vi "Parse RANGEFINDER.vi"(11 "Data":string) -> (2 "Voltage":sgl, 3 "Distance (m)":sgl)   [LabVIEW 2014]
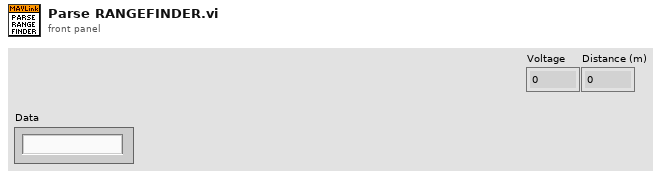
[diagram p1: front panel]
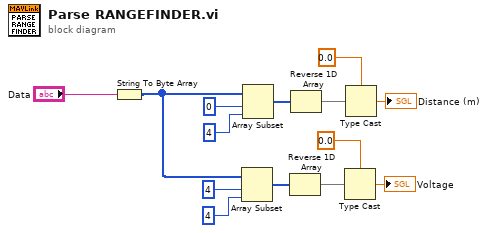
[diagram p0: block diagram]
diagram:
  n1 = String To Byte Array(string="Data") -> (unsigned byte array=w3:u8[])
  n2 = Array Subset(array=w3, index=4, length=4) -> (w5:u8[])
  n3 = Array Subset(array=w3, index=0, length=4) -> (w12:u8[])
  n4 = Reverse 1D Array(array=w5) -> (reversed array=w4:u8[])
  n5 = Reverse 1D Array(array=w12) -> (reversed array=w13:u8[])
  n6 = Type Cast(type=sgl 0.0 ("single precision float"), x=w4) -> (*(type *) &x=→"Voltage":sgl)
  n7 = Type Cast(type=sgl 0.0 ("single precision float"), x=w13) -> (*(type *) &x=→"Distance (m)":sgl)
